vi "DAQmx Create Channel (TEDS-AI-Strain-Strain Gage).vi"(0 "task in":refnum<k21>, 1 "maximum value":dbl=0.001 format="%0.7f", 2 "minimum value":dbl=-0.001 format="%0.7f", 5 "physical channels":tag, 7 "name to assign":string, 9 "units":i32(ring)=10299 items=["Strain"=10299, "From Custom Scale"=10065], 11 "error in":errorcluster, 12 "custom scale name":tag, 13 "bridge information":T1={"lead wire resistance"=0.0, "initial bridge voltage"=0.0, "voltage excitation source"=10200, "voltage excitation value"=2.5} {"initial bridge voltage" format="%0.2f"; "voltage excitation source" items=["Internal"=10200, "External"=10167, "None"=10230]; "voltage excitation value" format="%0.2f"; "lead wire resistance" format="%0.2f"}) -> (4 "task out":refnum<k21>, 15 "error out":errorcluster)   [LabVIEW 2020]
doc: "Creates channel(s) to measure strain. You must configure the physical channel(s) with TEDS information to use this VI."
uses:
  nilvaiu.dll
panel:
  # "input limits"
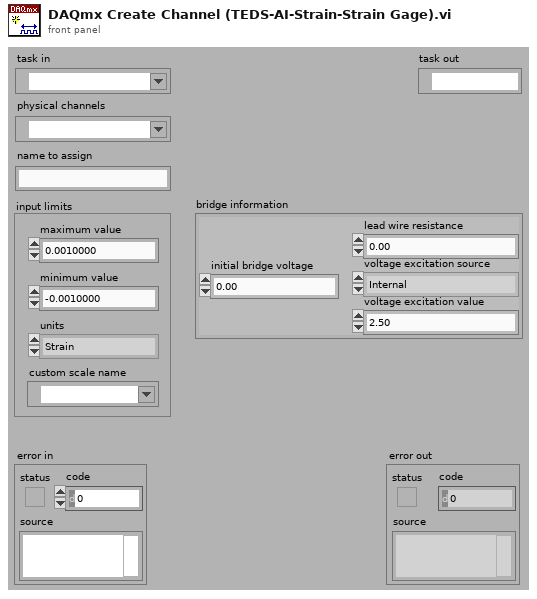
[diagram p1: front panel]
types:
  T1 = cluster{"lead wire resistance":dbl, "initial bridge voltage":dbl, "voltage excitation source":i32, "voltage excitation value":dbl}
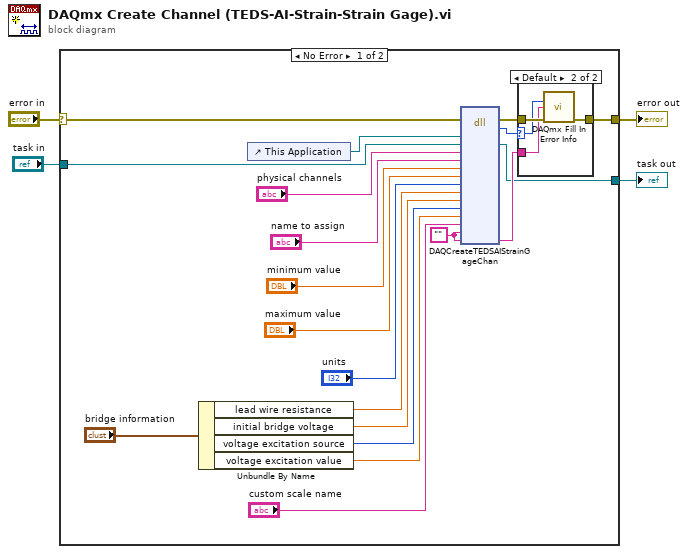
[diagram p0: block diagram]
diagram:
  n1 = case shown="No Error" "error in" {
    selector: "error in" -> [w19 w30]
    tunnel: [w22 w30] -> w4
    tunnel: "task in" -> [w8 w31]
    tunnel: [w6 w31] -> w1
    frame No Error {
      w5 = ""
      n2 = Unbundle By Name("bridge information") -> ("lead wire resistance"=w14:dbl, "initial bridge voltage"=w13:dbl, "voltage excitation source"=w12:i32, "voltage excitation value"=w11:dbl)
      n3 = control-ref of="This Application"() -> (w7:refnum<vi>)
      n4 = dll-call lib="nilvaiu.*" fn="DAQCreateTEDSAIStrainGageChan"(error in=w19, "lvAppRef"=w7, "refObjPtr"=w8, "physicalChannelName"="physical channels", "channelNameIn"="name to assign", "minVal"="minimum value", "maxVal"="maximum value", "units"="units", "leadWireResist"=w14, "initialBridgeVoltage"=w13, "excitSource"=w12, "excitValue"=w11, "customScaleName"="custom scale name", "channelNamesOut"=w5, "extendedErrorInfo"=w5) -> (error out=w23:errorcluster, "return type"=w20:i32, "refObjPtr"=w6:refnum<k21>, "extendedErrorInfo"=w21:string)  [unwired: 14 in, 1 out]
      n5 = case shown="Default" w20 {
        selector: w20 -> [_ w27]
        tunnel: w23 -> [w25 w29]
        tunnel: [w25 w28] -> w22
        tunnel: w21 -> [_ w26]
        frame 0 {
        }
        frame Default {
          n6 = call "DAQmx Fill In Error Info.vi"("status code"=w27, "extended error info"=w26, "error in"=w29) -> ("error out"=w28:errorcluster)  [unwired: 1 in, 11 out]
        }
      }
    }
    frame Error {
    }
  }
  "error out" <- w4
  "task out" <- w1
